vi "buffer - 2.vi"(8 "error in (no error)":errorcluster caption="エラー入力（エラーなし）", 9 "value in 2":dbl, 10 "value in":u32, 11 "FGV Mode":T1=enum."Get") -> (0 "error out":errorcluster caption="エラー出力", 1 "value out 2":dbl[](array[numeric]), 2 "value out":u32[](array[numeric]))   [LabVIEW 2018]
uses:
  FGV Mode.ctl
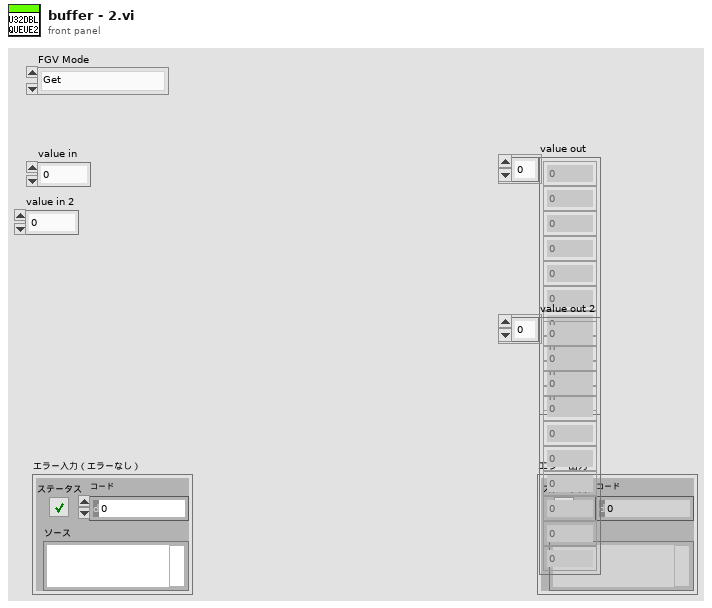
[diagram p1: front panel]
types:
  T1 = typedef "FGV Mode.ctl" = enum16{"None", "Init", "Set", "Get", "Update", "Clear"}
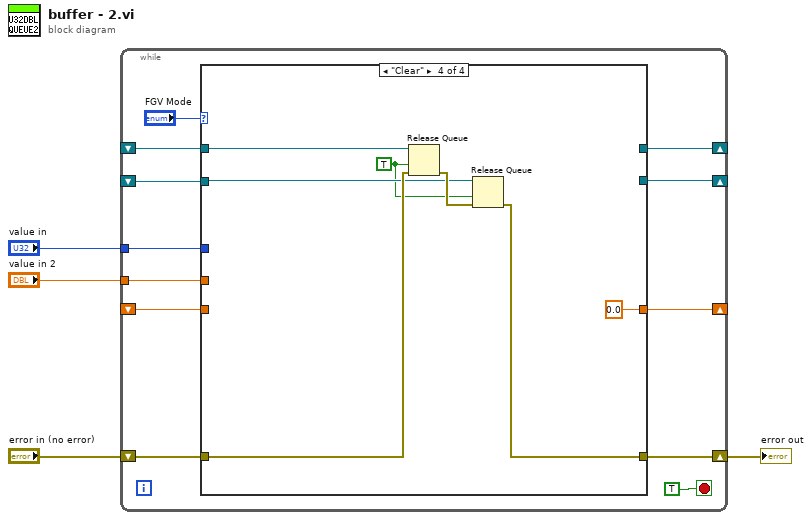
[diagram p0: block diagram]
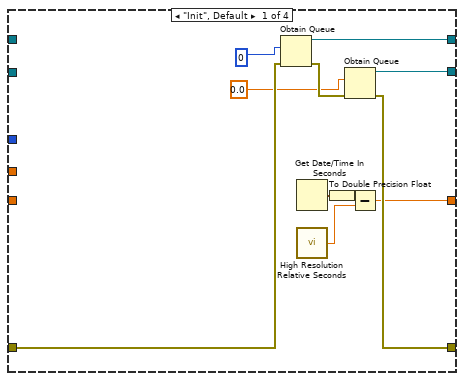
[diagram p2: hidden frame]
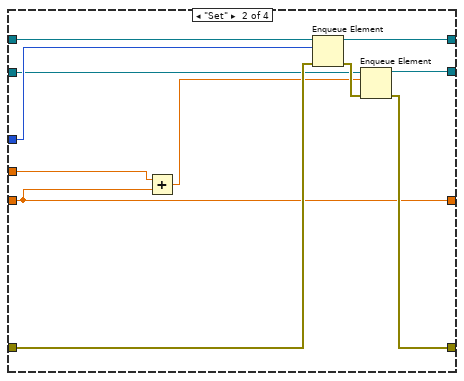
[diagram p3: hidden frame]
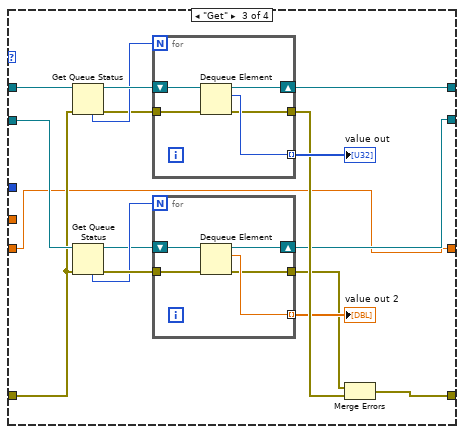
[diagram p4: hidden frame]
diagram:
  n1 = while {
    shift-right: [w14] -> w3
    shift-left: "error in (no error)" -> [w15]
    shift-right: [w12] -> _
    shift-left: _ -> [w11]
    tunnel: "value in" -> [w10]
    shift-right: [w9] -> _
    shift-left: _ -> [w8]
    tunnel: "value in 2" -> [w7]
    shift-right: [w6] -> _
    shift-left: _ -> [w5]
    stop <- TRUE stop-if-true
    n2 = case shown="\"Clear\"" "FGV Mode" {
      tunnel: w15 -> [w25 w35 w43 w71]
      tunnel: [w23 w33 w41 w67] -> w14
      tunnel: [w27 w37 w55 _] -> w12
      tunnel: w11 -> [_ w38 w54 w72]
      tunnel: w10 -> [_ w36 _ _]
      tunnel: [w22 w32 w42 _] -> w9
      tunnel: w8 -> [_ w31 w44 w69]
      tunnel: w7 -> [_ w30 _ _]
      tunnel: [w18 w28 w39 0.0] -> w6
      tunnel: w5 -> [_ w28 w39 _]
      frame "Init", Default {
        n3 = Obtain Queue(element data type=u32 0 ("Elements Remaining"), error in (no error)=w25) -> (queue out=w27:refnum<queue>, error out=w24:errorcluster)  [unwired: 3 in, 1 out]
        n4 = Get Date/Time In Seconds() -> (seconds since 1Jan1904=w20:timestamp)
        n5 = call <vilib>:"High Resolution Relative Seconds.vi"() -> ("relative seconds"=w19:dbl)
        n6 = To Double Precision Float(number=w20) -> (double precision float=w17:dbl)
        n7 = Obtain Queue(element data type=0.0 ("Elements Remaining"), error in (no error)=w24) -> (queue out=w22:refnum<queue>, error out=w23:errorcluster)  [unwired: 3 in, 1 out]
        n8 = Subtract(x=w17, y=w19) -> (x-y=w18:dbl)
      }
      frame "Set" {
        n9 = Add(x=w30, y=w28) -> (x+y=w29:dbl)
        n10 = Enqueue Element(queue=w38, element=w36, error in (no error)=w35) -> (queue out=w37:refnum<queue>, error out=w34:errorcluster)  [unwired: 1 in, 1 out]
        n11 = Enqueue Element(queue=w31, element=w29, error in (no error)=w34) -> (queue out=w32:refnum<queue>, error out=w33:errorcluster)  [unwired: 1 in, 1 out]
      }
      frame "Get" {
        n12 = Get Queue Status(queue=w54, error in (no error)=w43) -> (queue out=w53:refnum<queue>, error out=w49:errorcluster, # elements in queue=w52:i32)  [unwired: 1 in, 5 out]
        n13 = Get Queue Status(queue=w44, error in (no error)=w43) -> (queue out=w45:refnum<queue>, error out=w48:errorcluster, # elements in queue=w46:i32)  [unwired: 1 in, 5 out]
        n14 = for {
          N: w52 -> [_]
          shift-right: [w65] -> w55
          shift-left: w53 -> [w64]
          tunnel: [w63] -> w51 mode=indexing
          tunnel: w49 -> [w62]
          tunnel: [w61] -> w50
          n15 = Dequeue Element(queue=w64, error in (no error)=w62) -> (queue out=w65:refnum<queue>, element=w63:u32, error out=w61:errorcluster)  [unwired: 1 in, 1 out]
        }
        "value out" <- w51
        n16 = for {
          N: w46 -> [_]
          shift-right: [w60] -> w42
          shift-left: w45 -> [w59]
          tunnel: [w58] -> w47 mode=indexing
          tunnel: w48 -> [w57]
          tunnel: [w56] -> w40
          n17 = Dequeue Element(queue=w59, error in (no error)=w57) -> (queue out=w60:refnum<queue>, element=w58:dbl, error out=w56:errorcluster)  [unwired: 1 in, 1 out]
        }
        "value out 2" <- w47
        n18 = Merge Errors(w40, w50) -> (w41:errorcluster)
      }
      frame "Clear" {
        w68 = TRUE ("破棄を強制? (F)")
        n19 = Release Queue(queue=w72, force destroy? (F)=w68, error in (no error)=w71) -> (error out=w70:errorcluster)  [unwired: 2 out]
        n20 = Release Queue(queue=w69, force destroy? (F)=w68, error in (no error)=w70) -> (error out=w67:errorcluster)  [unwired: 2 out]
      }
    }
  }
  "error out" <- w3
